vi "Calculate motion steps.vi"(8 "error in (no error)":errorcluster, 11 "ConfocalStage in":refnum<class "ConfocalStage.lvclass">) -> (0 "error out":errorcluster, 2 "Relative motion array":dbl[](array[numeric]), 3 "ConfocalStage out":refnum<class "ConfocalStage.lvclass">)   [LabVIEW 2012, in "ConfocalStage.lvclass"]
uses:
  ConfocalStage.lvclass
  ConfocalStage.lvclass/ConfocalStage.ctl
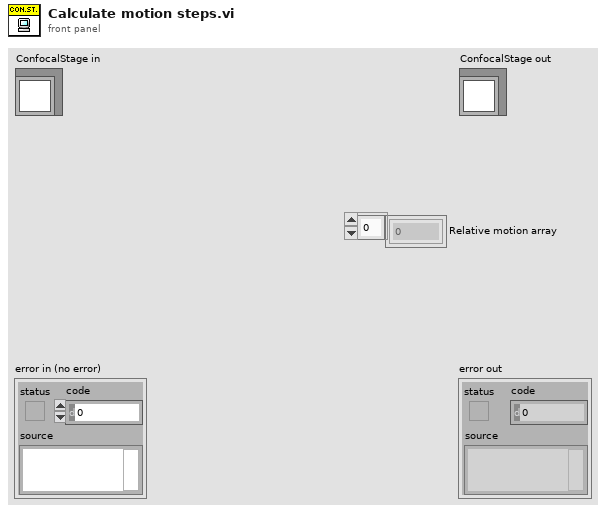
[diagram p1: front panel]
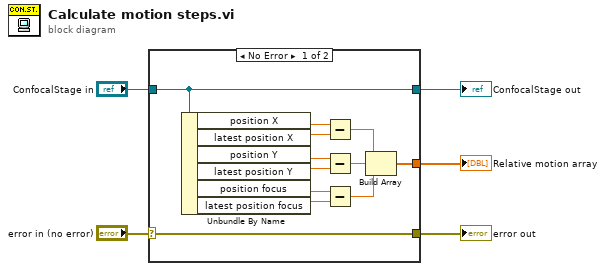
[diagram p0: block diagram]
diagram:
  n1 = case shown="No Error" "error in (no error)" {
    selector: "error in (no error)" -> [w17 w19]
    tunnel: [w17 w19] -> w4
    tunnel: [w16 w18] -> w2
    tunnel: "ConfocalStage in" -> [w16 w18]
    tunnel: [w6 _] -> w1
    frame No Error {
      n2 = Unbundle By Name(w16) -> ("position X"=w15:dbl, "latest position X"=w14:dbl, "position Y"=w13:dbl, "latest position Y"=w12:dbl, "position focus"=w11:dbl, "latest position focus"=w10:dbl)
      n3 = Subtract(x=w15, y=w14) -> (x-y=w9:dbl)
      n4 = Subtract(x=w13, y=w12) -> (x-y=w8:dbl)
      n5 = Subtract(x=w11, y=w10) -> (x-y=w7:dbl)
      n6 = Build Array(w9, w8, w7) -> (w6:dbl[])
    }
    frame Error {
    }
  }
  "error out" <- w4
  "ConfocalStage out" <- w2
  "Relative motion array" <- w1
